vi "Theme4_Topic4_qn8.vi"(9 "RefPrevious":refnum<vi>, 10 "RefNext":refnum<vi>, 11 "connection reference":T1) -> (2 "AnsIndicator":refnum<vi>[](array[refnum]))   [LabVIEW 2013]
uses:
  why.vi
  Precontrol.vi
  <vilib>/addons/database/Connection.llb/Conn ObjectReference.ctl
  <vilib>/addons/database/NI_Database_API.lvlib
panel:
  out "Why?":string
  out "Header":string[][](table)
  out "MCQ_RandomizedTbl":string[][](table)
  out "DInd":bool
  out "CInd":bool
  out "BInd":bool
  out "AInd":bool
  in  "ABCD":enum32{"No Selection", "A", "B", "C", "D"}(radio)
  # "Which of the following about sound waves is correct?"
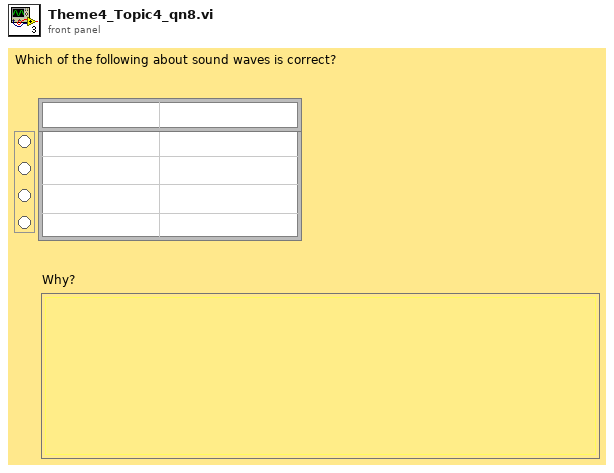
[diagram p1: front panel]
types:
  T1 = typedef "NI_Database_API.lvlib/Conn ObjectReference.ctl" = refnum<k1>
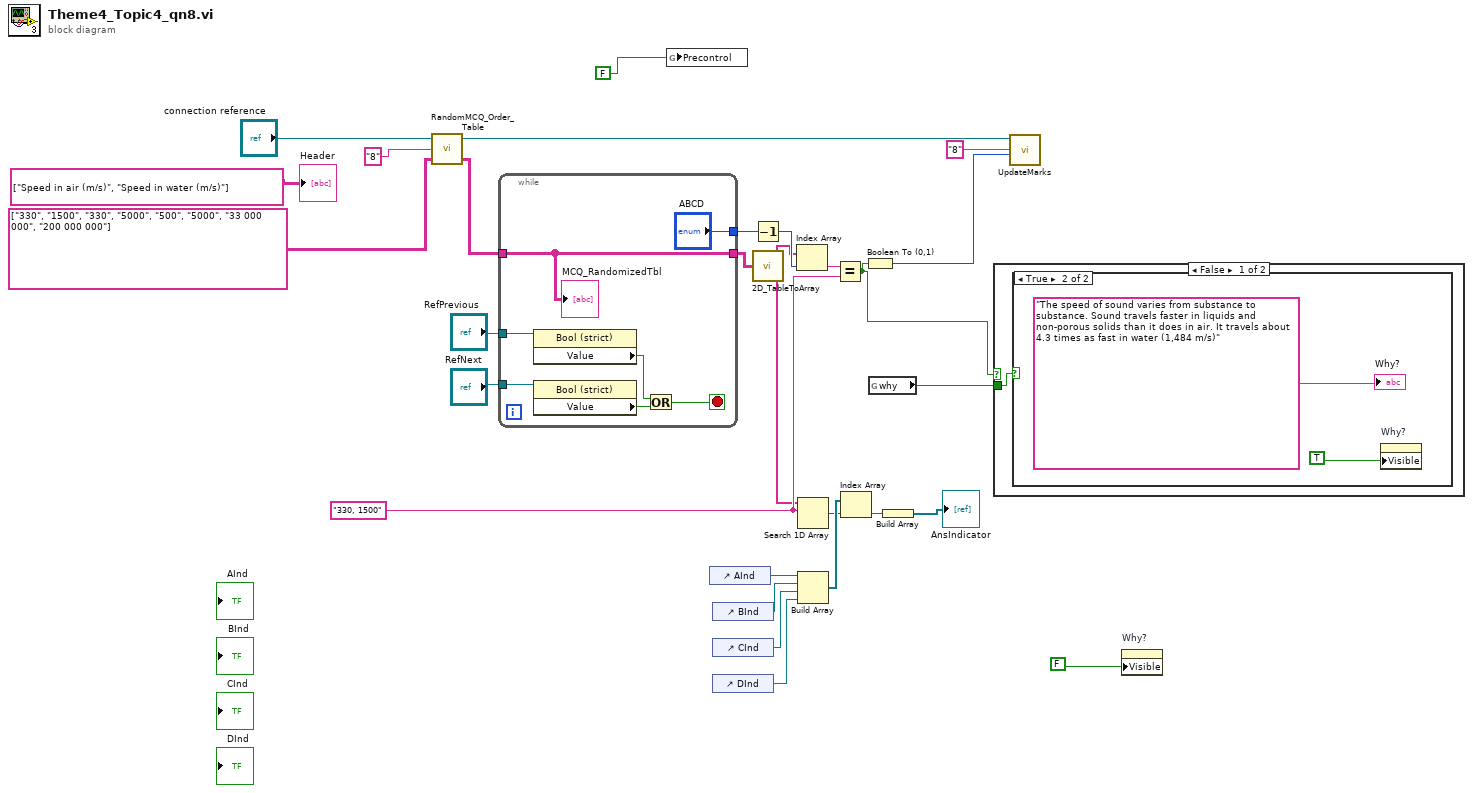
[diagram p0: block diagram]
diagram:
  w10 = "330, 1500" ("element")
  n1 = call "RandomMCQ_Order_Table.vi"("MCQ_Ordered"=string[][] [["330", "1500"], ["330", "5000"], ["500", "5000"], ["33 000 000", "200 000 000"]] ("MCQ_Randomized"), "Questions_Ordered"="8", "connection reference"="connection reference") -> ("MCQ_Randomized"=w28:string[][], "connection reference out"=w15:T1)  [unwired: 1 in]
  n2 = while {
    tunnel: ["ABCD"] -> w2
    tunnel: w28 -> [w29]
    tunnel: [w29] -> w11
    tunnel: "RefNext" -> [w31]
    tunnel: "RefPrevious" -> [w32]
    stop <- w30 stop-if-true
    n3 = property class="Bool (strict)"(reference=w32) -> ("Value"=w34:bool)  [unwired: 1 in, 2 out]
    n4 = property class="Bool (strict)"(reference=w31) -> ("Value"=w33:bool)  [unwired: 1 in, 2 out]
    n5 = Or(x=w34, y=w33) -> (x .or. y?=w30:bool)
    "MCQ_RandomizedTbl" <- w29
  }
  n6 = global write "Precontrol.vi" "Precontrol"(FALSE) -> ()
  n7 = control-ref of="AInd"() -> (w25:refnum<vi>)
  n8 = control-ref of="BInd"() -> (w24:refnum<vi>)
  n9 = control-ref of="CInd"() -> (w23:refnum<vi>)
  n10 = control-ref of="DInd"() -> (w22:refnum<vi>)
  n11 = Decrement(x=w2) -> (x-1=w12:enum32{"No Selection", "A", "B", "C", "D"})
  n12 = call "2D_TableToArray.vi"("TableIn"=w11) -> ("\"col1\", \"col2\""=w9:string[])
  n13 = Index Array(array=w9, index=w12) -> (element=w18:string)
  n14 = Search 1D Array(1D array=w9, element=w10) -> (index of element=w20:i32)  [unwired: 1 in]
  n15 = Build Array(w25, w24, w23, w22) -> (w21:refnum<vi>[])
  n16 = Equal?(x=w18, y=w10) -> (x = y?=w5:bool)
  n17 = Index Array(array=w21, index=w20) -> (element=w19:refnum<vi>)
  n18 = Boolean To (0,1)(Boolean=w5) -> (0, 1=w6:i16)
  n19 = global read "why.vi" "why"() -> (w4:bool)
  n20 = Build Array(w19) -> (→"AnsIndicator":refnum<vi>[])
  n21 = case shown="False" w5 {
    tunnel: w4 -> [w36 _]
    frame False {
      n22 = case shown="True" w36 {
        frame False {
        }
        frame True {
          n23 = property on="Why?" class="Str"("Visible"=TRUE) -> ()  [unwired: 2 in, 2 out]
          "Why?" <- "The speed of sound varies from substance to substance. Sound travels faster in liquids and non-porous solids than it does in air. It travels about 4.3 times as fast in water (1,484 m/s)"
        }
      }
    }
    frame True {
    }
  }
  n24 = call "UpdateMarks.vi"("MarksEarned"=w6, "QuestionsNo_Ordered"="8", "connection reference"=w15) -> ()  [unwired: 9 in]
  n25 = property on="Why?" class="Str"("Visible"=FALSE) -> ()  [unwired: 2 in, 2 out]
  "Header" <- string[][] [["Speed in air (m/s)", "Speed in water (m/s)"]] ("MCQ_Randomized")
